vi "Read Channel Info.vi"(8 "error in (no error)":errorcluster, 11 "Dummy.lvclass in":refnum<class "Dummy.lvclass">) -> (0 "error out":errorcluster, 1 "Channel Units":string[](array[string]), 2 "Channel Names":string[](array[string]), 3 "Dummy.lvclass out":refnum<class "Dummy.lvclass">, 5 "#Channels":i32)   [LabVIEW 2009, in "Dummy.lvclass"]
doc: "(Dynamic) Return information about the readable data channels this object provides, e.g., the name of each data source and its unit."
uses:
  Dummy.lvclass
  Readable/Readable.lvclass
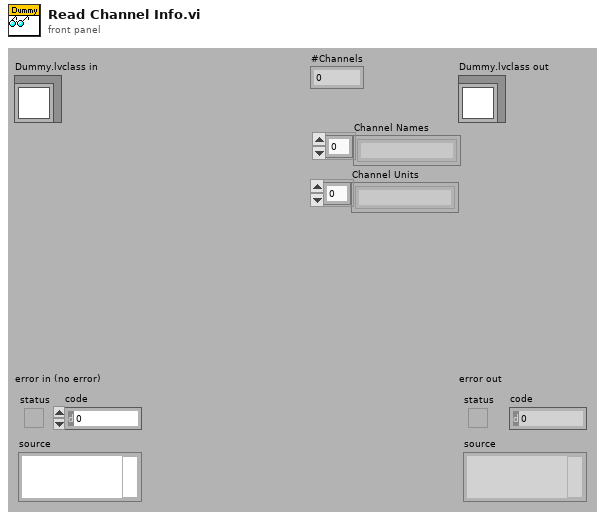
[diagram p1: front panel]
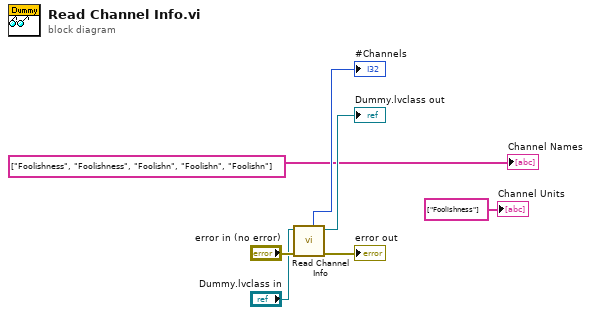
[diagram p0: block diagram]
diagram:
  n1 = call-parent "Read Channel Info.vi"("error in (no error)"="error in (no error)", "Readable.lvclass in"="Dummy.lvclass in") -> ("error out"=→"error out":errorcluster, "Readable.lvclass out"=→"Dummy.lvclass out":refnum<class "Dummy.lvclass">, "#Channels"=→"#Channels":i32)  [unwired: 5 in, 2 out]
  "Channel Units" <- string[] ["Foolishness"] ("Channel Units")
  "Channel Names" <- string[] ["Foolishness", "Foolishness", "Foolishn", "Foolishn", "Foolishn"] ("Channel Names")
